vi "ResetAlarm.vi"(10 "reset":bool, 11 "Sig_AI in":refnum<class "Sig_AI.lvclass">) -> (3 "Sig_AI out":refnum<class "Sig_AI.lvclass">)   [LabVIEW 2019, in "Sig_AI.lvclass"]
uses:
  Sig_AI.lvclass
  Sig_AI.lvclass/Sig_AI.ctl
  AnalogComparator_class/AnalogComparator.lvclass/AnalogComparator.ctl
  AnalogComparator_class/AnalogComparator.lvclass
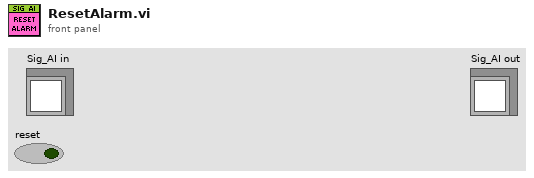
[diagram p1: front panel]
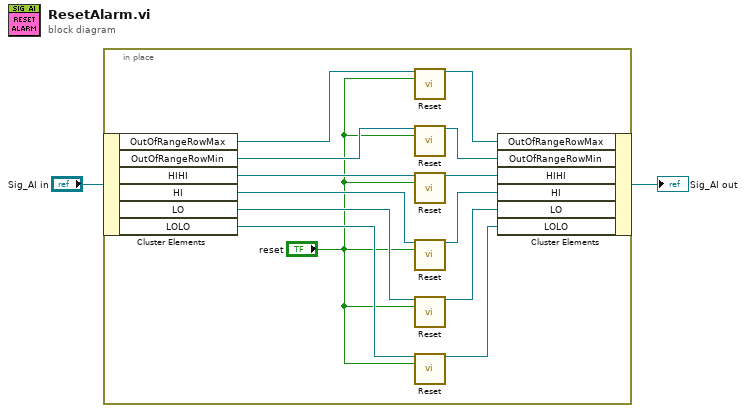
[diagram p0: block diagram]
diagram:
  n1 = in-place {
    n2 = in-place-cluster #1("Sig_AI in") -> ("OutOfRangeRowMax"=w15:refnum<class "AnalogComparator.lvclass">, "OutOfRangeRowMin"=w13:refnum<class "AnalogComparator.lvclass">, "HIHI"=w12:refnum<class "AnalogComparator.lvclass">, "HI"=w11:refnum<class "AnalogComparator.lvclass">, "LO"=w10:refnum<class "AnalogComparator.lvclass">, "LOLO"=w9:refnum<class "AnalogComparator.lvclass">)
    n3 = call "Reset.vi"("class data in"=w15, "reset"="reset") -> ("class data out"=w14:refnum<class "AnalogComparator.lvclass">)  [unwired: 13 in]
    n4 = call "Reset.vi"("class data in"=w13, "reset"="reset") -> ("class data out"=w8:refnum<class "AnalogComparator.lvclass">)  [unwired: 13 in]
    n5 = call "Reset.vi"("class data in"=w12, "reset"="reset") -> ("class data out"=w7:refnum<class "AnalogComparator.lvclass">)  [unwired: 13 in]
    n6 = call "Reset.vi"("class data in"=w11, "reset"="reset") -> ("class data out"=w6:refnum<class "AnalogComparator.lvclass">)  [unwired: 13 in]
    n7 = call "Reset.vi"("class data in"=w10, "reset"="reset") -> ("class data out"=w5:refnum<class "AnalogComparator.lvclass">)  [unwired: 13 in]
    n8 = call "Reset.vi"("class data in"=w9, "reset"="reset") -> ("class data out"=w4:refnum<class "AnalogComparator.lvclass">)  [unwired: 13 in]
    n9 = in-place-cluster #1("OutOfRangeRowMax"=w14, "OutOfRangeRowMin"=w8, "HIHI"=w7, "HI"=w6, "LO"=w5, "LOLO"=w4) -> (→"Sig_AI out":refnum<class "Sig_AI.lvclass">)
  }
